vi "Process.vi"(8 "error in":errorcluster, 11 "Example Instrument":refnum<class "Instrument.FrameworkTemplate.lvclass">) -> (0 "error out":errorcluster, 3 "Example Instrument out":refnum<class "Instrument.FrameworkTemplate.lvclass">)   [LabVIEW 2019, in "Instrument.FrameworkTemplate.lvclass"]
doc: "---------------------------------------------------------------\nJKI State Machine Objects™\nhttp://jki.net/state-machine-objects/\nCopyright (C) 2005-2015, JKI <info@jki.net>\nALL RIGHTS RESERVED"
uses:
  Instrument.FrameworkTemplate.lvclass
  C:/Program Files (x86)/National Instruments/LabVIEW 2019/vi.lib/JKI/JKI SMO/SMO/SMO.lvclass
  <vilib>/JKI/JKI SMO/SMO/SMO.lvclass/SMO.ctl
  <vilib>/JKI/JKI SMO/SMO/Private/ReftoDVR--SMO.vi
  <userlib>/LevyLab/Instrument Framework/Instrument Types/VSource/Instrument.VSource.lvclass
  <vilib>/JKI/JKI SMO/SMO/SMO.lvclass
panel:
  # "Example INSTRUMENT"
  # "For instructions on how to use the JKI State Machine Objects, examples and video tutorials, visit:\nhttp://jki.net/state-machine-objects/\n\nJKI State Machine Objects™\nhttp://jki.net/state-machine-objects/\nCopyright (C) 2005-2015, JKI <info@jki.net>\nALL RIGHTS RESERVED"
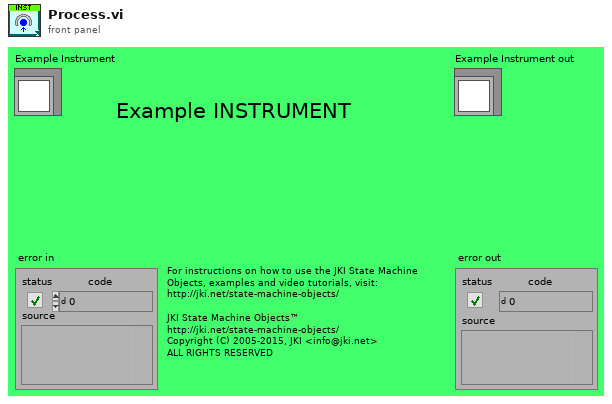
[diagram p1: front panel]
types:
  T1 = enum32{"invalid app kind", "Development System", "Run Time System", "Student Edition", "Embedded LabVIEW", "Evaluation", "Custom"}
  T2 = enum32{"Invalid", "Standard", "Closed", "Hidden", "Minimized", "Maximized"}
  T3 = enum32{"Bad", "Idle", "Run top level", "Running"}
  T4 = cluster{"Core":cluster{"Current VI Reference":refnum<vi>, "Close Panel on Exit?":bool, "error":errorcluster}, "Self Reference":refnum<class "Instrument.FrameworkTemplate.lvclass">}
  T5 = cluster{"Current VI Reference":refnum<vi>, "Close Panel on Exit?":bool, "error":errorcluster}
  T6 = typedef "SMO.lvclass/Protected Events.ctl" = cluster{"StopProcesses":refnum<user-event>, "AbortProcesses":refnum<user-event>, "Config Changed":refnum<user-event>, "Dependency":refnum<user-event>}
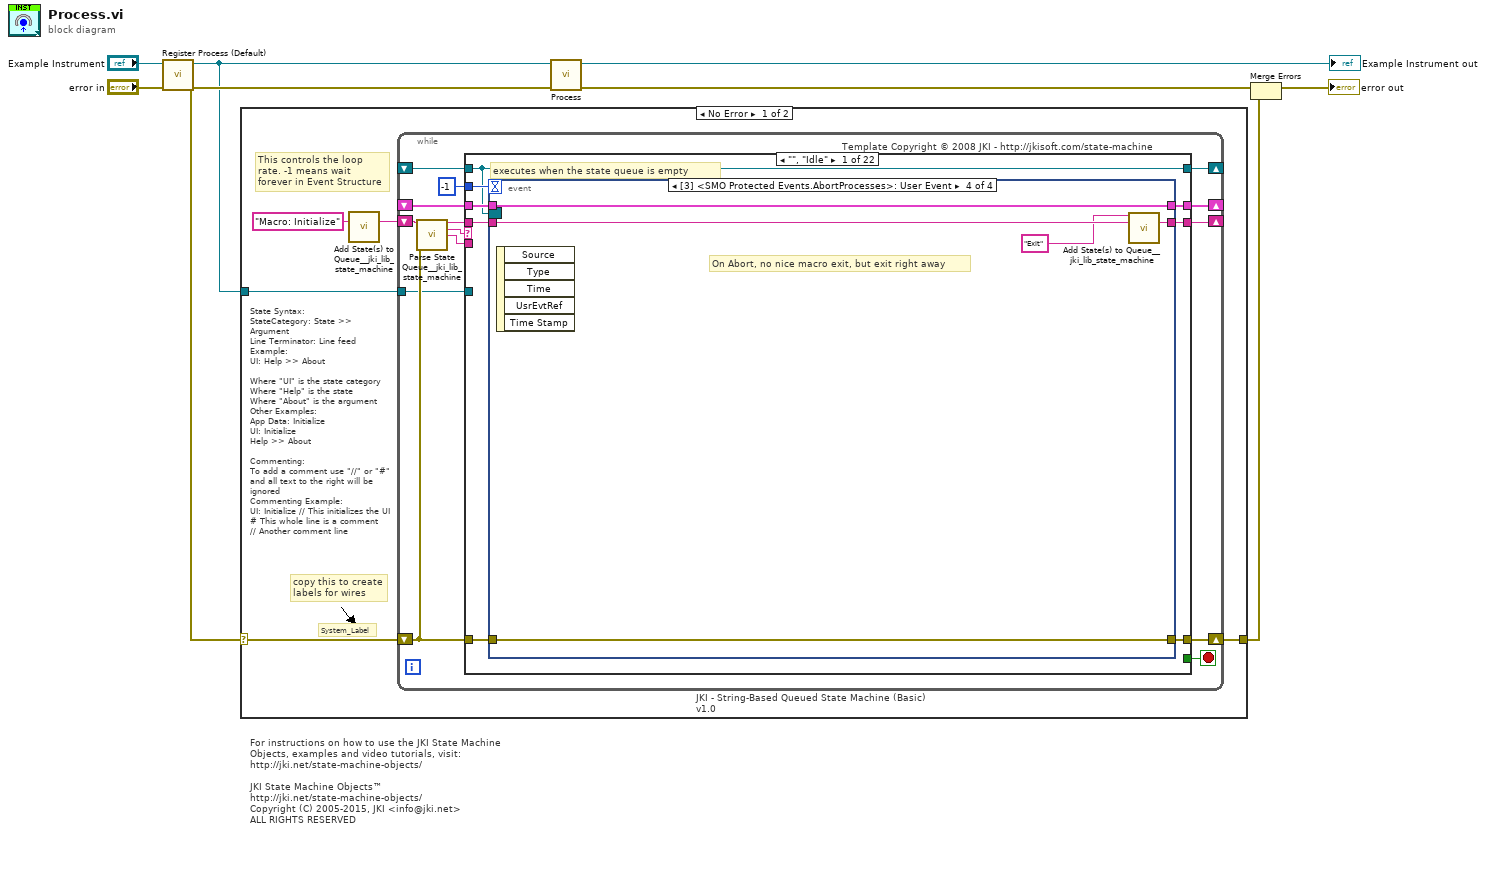
[diagram p0: block diagram]
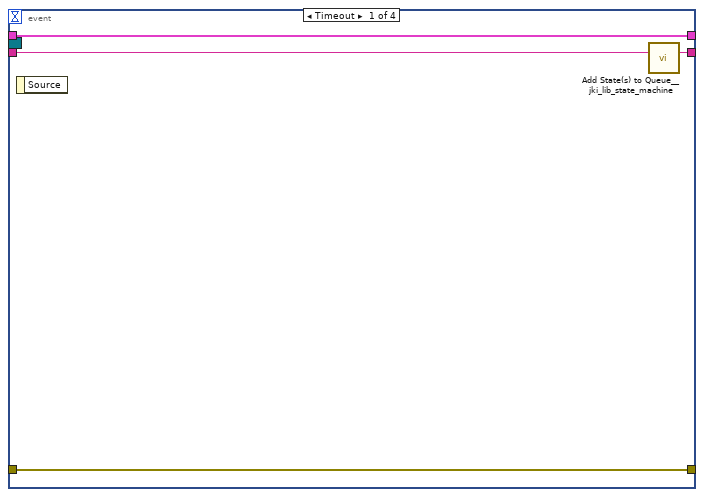
[diagram p2: hidden frame]
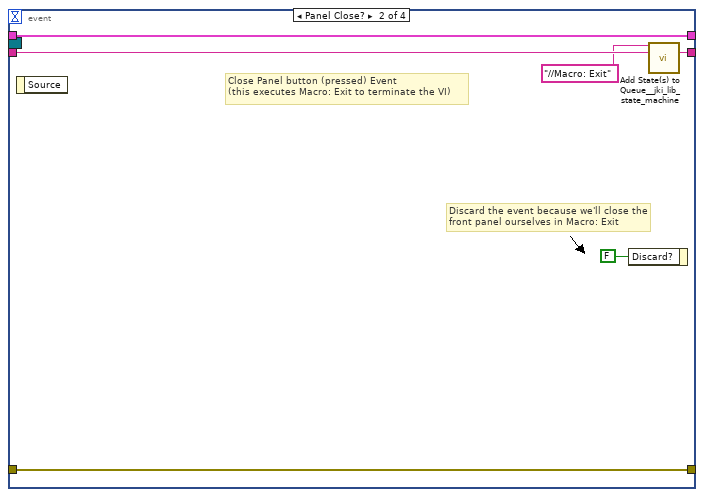
[diagram p3: hidden frame]
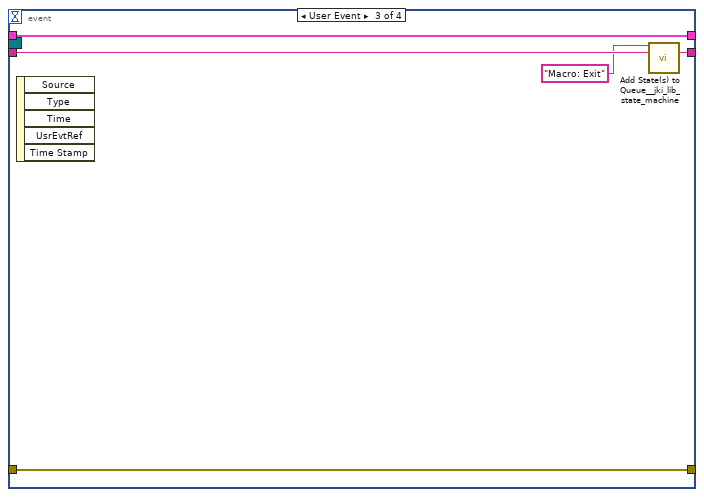
[diagram p4: hidden frame]
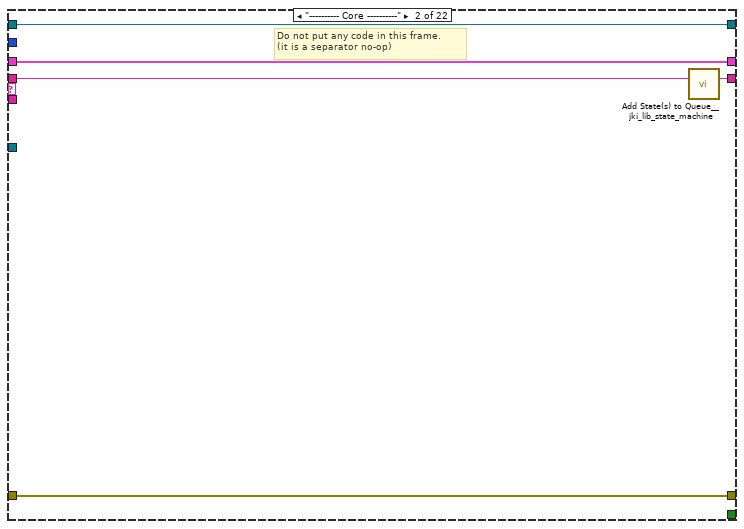
[diagram p5: hidden frame]
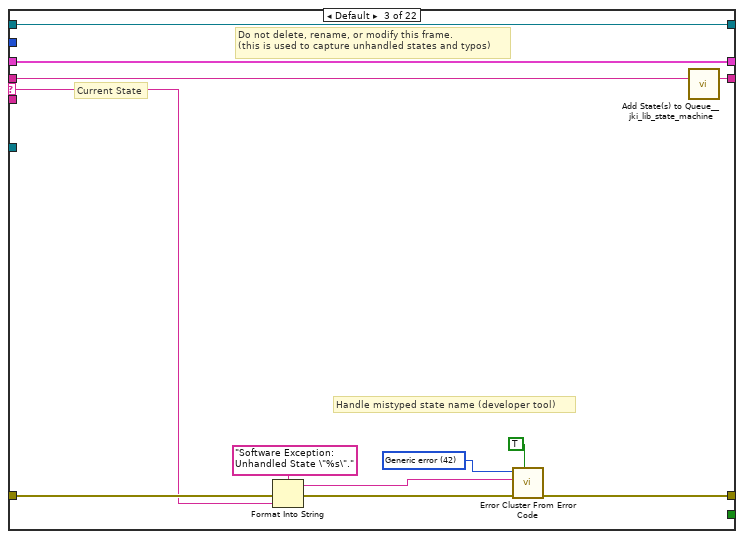
[diagram p6: hidden frame]
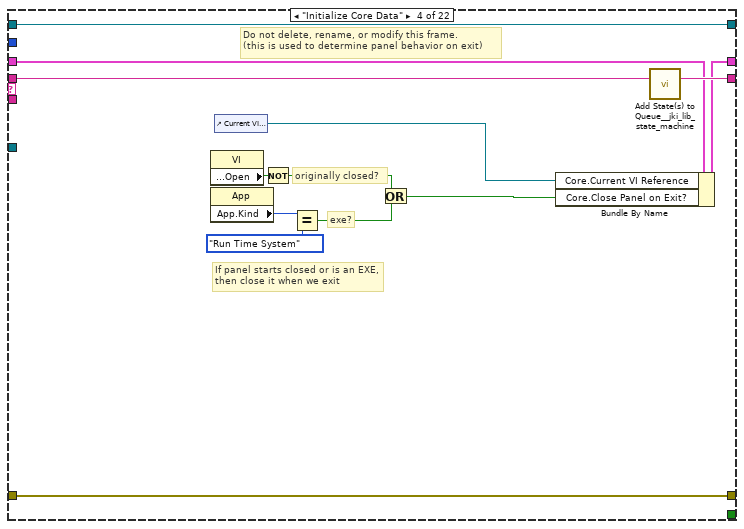
[diagram p7: hidden frame]
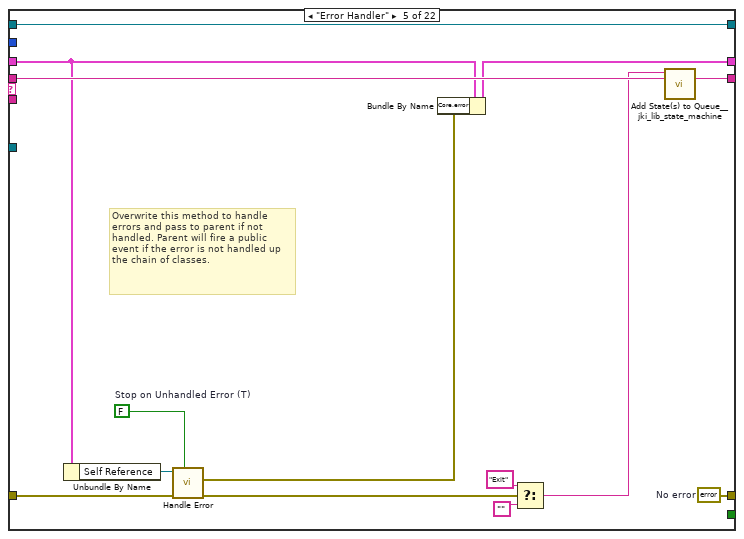
[diagram p8: hidden frame]
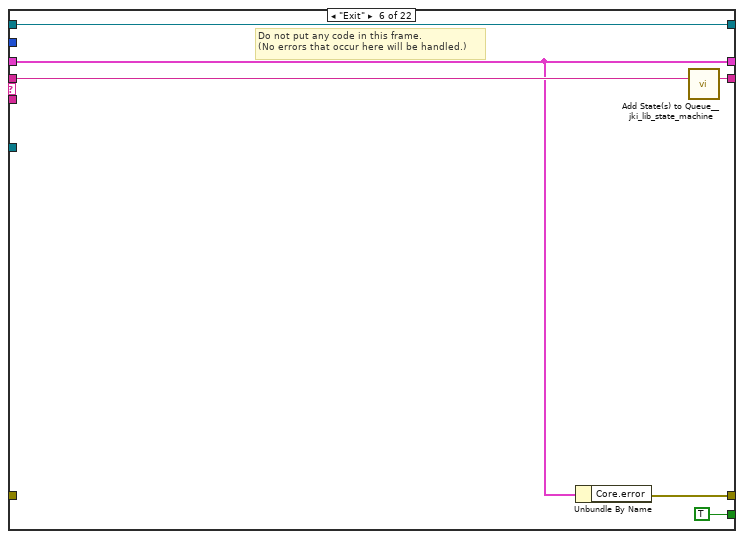
[diagram p9: hidden frame]
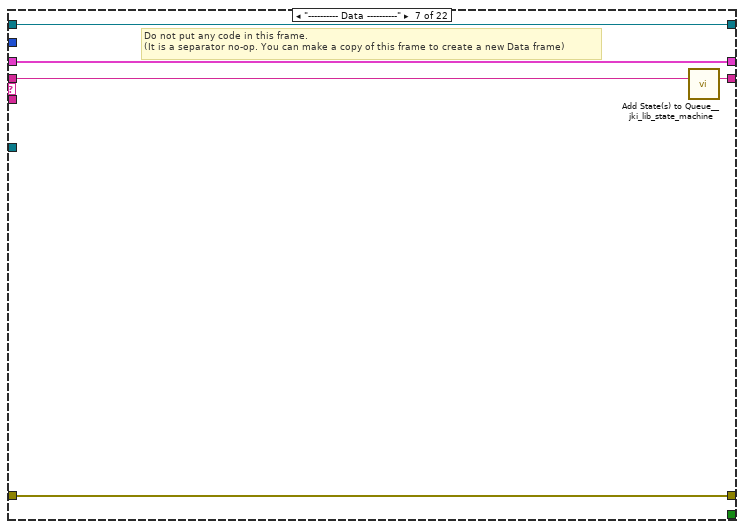
[diagram p10: hidden frame]
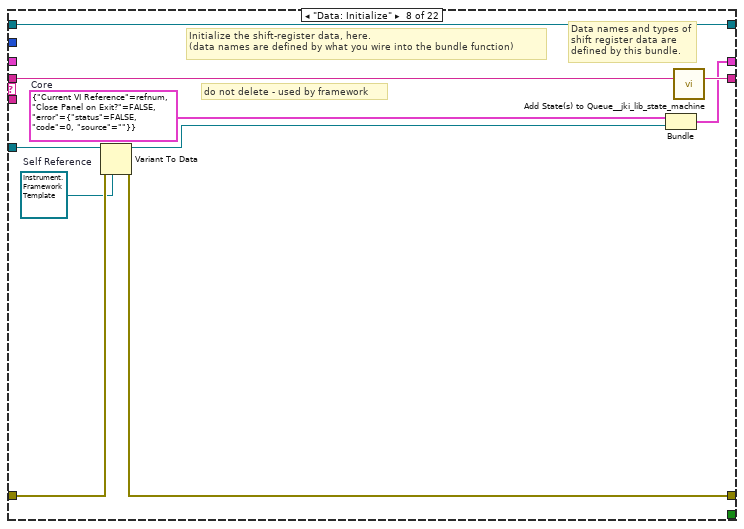
[diagram p11: hidden frame]
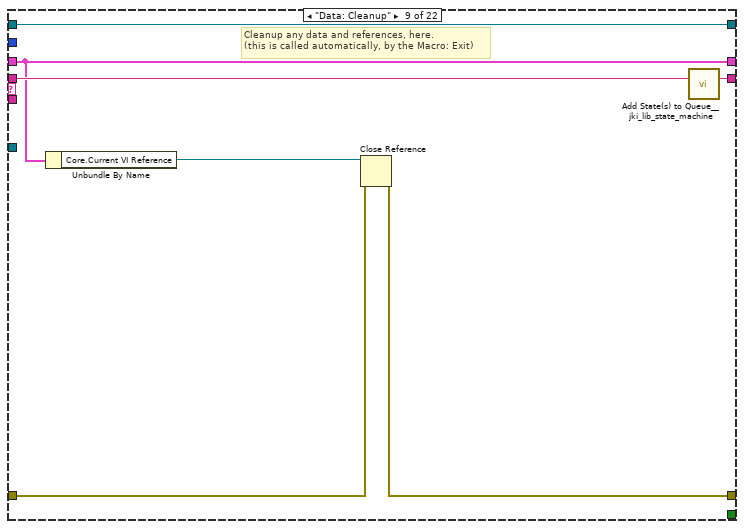
[diagram p12: hidden frame]
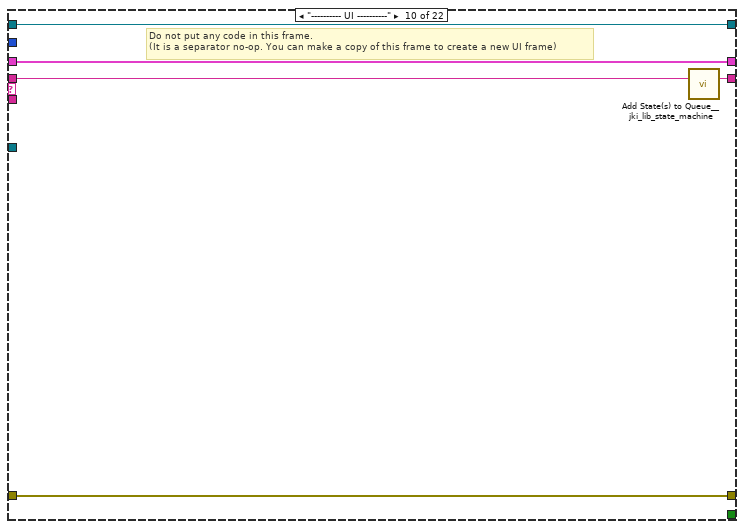
[diagram p13: hidden frame]
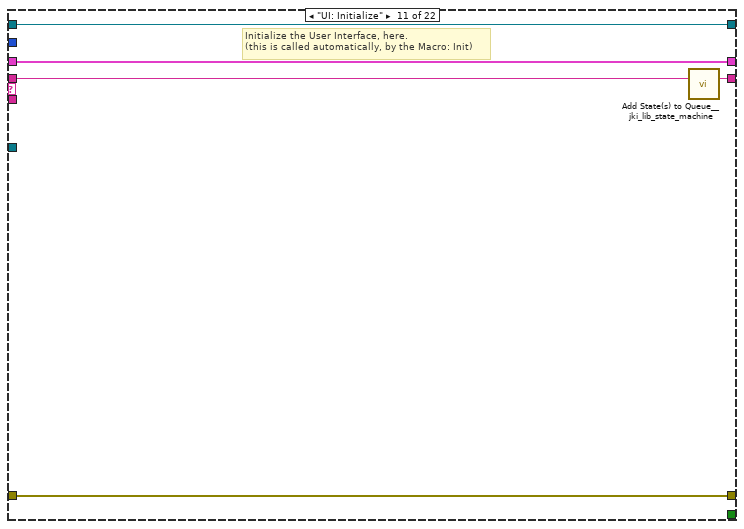
[diagram p14: hidden frame]
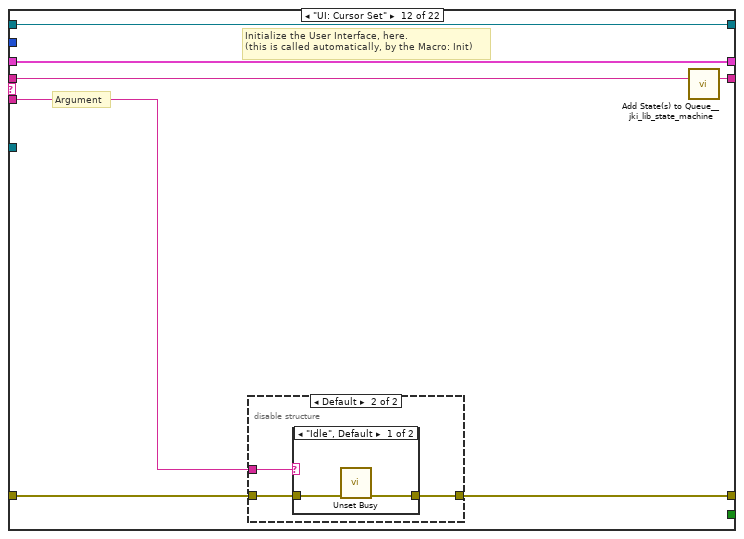
[diagram p15: hidden frame]
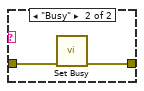
[diagram p17: hidden frame]
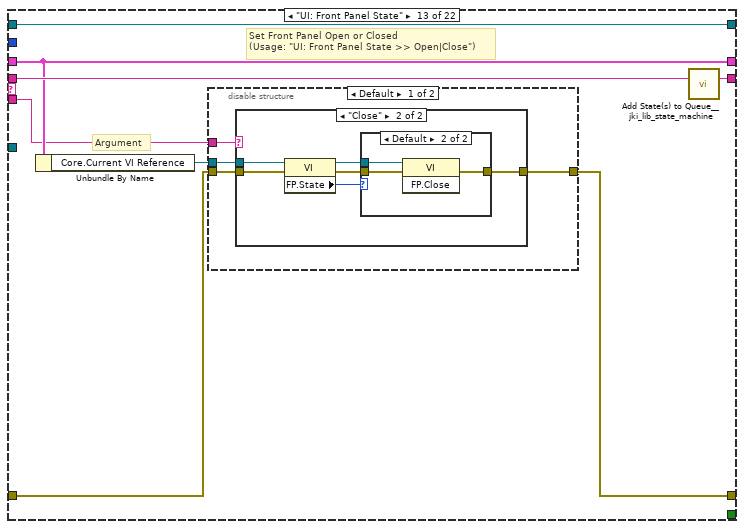
[diagram p18: hidden frame]
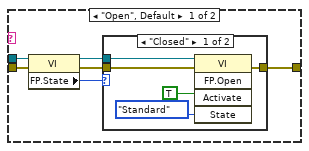
[diagram p19: hidden frame]
diagram:
  # "For instructions on how to use the JKI State Machine Objects, examples and video tutorials, visit:\nhttp://jki.net/state-machine-objects/\n\nJKI State Machine Objects™\nhttp://jki.net/state-machine-objects/\nCopyright (C) 2005-2015, JKI <info@jki.net>\nALL RIGHTS RESERVED"
  n1 = call <vilib>:"Register Process (Default).vi"("error in (no error)"="error in", "SMO"="Example Instrument") -> ("error out"=w5:errorcluster, "SelfRef"=w4:refnum<class "Instrument.FrameworkTemplate.lvclass">)  [unwired: 8 in]
  n2 = case shown="No Error" w5 {
    selector: w5 -> [w10 w279]
    tunnel: w4 -> [w11 _]
    tunnel: [w9 w279] -> w1
    frame No Error {
      # "State Syntax:\nStateCategory: State >> Argument\nLine Terminator: Line feed\nExample:\nUI: Help >> About\n\nWhere \"UI\" is the state category\nWhere \"Help\" is the state\nWhere \"About\" is the argument\nOther Examples:\nApp Data: Initialize\nUI: Initialize\nHelp >> About\n\nCommenting:\nTo add a comment use \"//\" or \"#\" and all text to the right will be ignored\nCommenting Example:\nUI: Initialize // This initializes the UI\n# This whole line is a comment\n// Another comment line"
      # "copy this to create labels for wires"
      # "This controls the loop rate. -1 means wait forever in Event Structure"
      # "System_Label"
      n3 = call <vilib>:"Add State(s) to Queue__jki_lib_state_machine.vi"("State(s) in (\"\")"="Macro: Initialize") -> ("States Out"=w13:string)  [unwired: 14 in]
      n4 = while "JKI - String-Based Queued State Machine (Basic) v1.0" {
        shift-right: [w20] -> _
        shift-left: _ -> [w19]
        shift-right: [w23] -> w9
        shift-left: w10 -> [w17]
        shift-right: [w22] -> _
        shift-left: w13 -> [w24]
        tunnel: w11 -> [w16]
        shift-right: [w15] -> _
        shift-left: _ -> [w14]
        stop <- w21 stop-if-true
        # "Template Copyright © 2008 JKI - http://jkisoft.com/state-machine"
        n5 = call <vilib>:"Parse State Queue__jki_lib_state_machine.vi"("State Queue"=w24, "Error In (no error)"=w17) -> ("Remaining States"=w26:string, "Current State"=w27:string, "Arguments"=w25:string)  [unwired: 11 in]
        n6 = case shown="\"\", \"Idle\"" w27 {
          selector: w27 -> [_ _ w62 _ _ _ _ _ _ _ _ _ _ _ _ _ _ _ _ _ _ _]
          tunnel: w26 -> [w35 w60 w66 w85 w99 w105 w110 w120 w127 w132 w137 w144 w160 w192 w215 w236 w241 w252 w257 w267 w273 w278]
          tunnel: w25 -> [_ _ _ _ _ _ _ _ _ _ _ w138 w154 _ _ _ _ _ _ _ _ _]
          tunnel: w19 -> [w33 w57 w64 w76 w93 w101 w107 _ w122 w129 w135 w142 w156 w189 w212 w217 w238 w249 w254 w258 w271 w276]
          tunnel: [w32 w58 w68 w82 w94 w100 w108 w111 w123 w130 w134 w139 w157 w190 w194 w219 w239 w243 w255 w262 w269 w274] -> w23
          tunnel: w17 -> [w31 w58 w67 w82 w95 _ w108 w117 w124 w130 w134 w140 w158 w190 w195 w220 w239 w244 w255 w263 w269 w274]
          tunnel: [w34 w59 w65 w84 w98 w104 w109 w119 w126 w131 w136 w143 w159 w191 w214 w235 w240 w251 w256 w266 w272 w277] -> w22
          tunnel: [_ _ _ _ _ TRUE _ _ _ _ _ _ _ _ _ _ _ _ _ _ _ _] -> w21
          tunnel: [w30 w57 w64 w83 w92 w101 w107 w118 w122 w129 w135 w142 w156 w189 w212 w217 w238 w249 w254 w258 w271 w276] -> w20
          tunnel: -1 ("Timeout") -> [w29 _ _ _ _ _ _ _ _ _ _ _ _ _ _ _ _ _ _ _ _ _]
          tunnel: w16 -> [_ _ _ _ _ _ _ w115 _ _ _ _ _ _ w203 w216 _ _ _ _ _ _]
          tunnel: [w28 w56 w61 w73 w97 w102 w106 w114 w121 w128 w133 w141 w153 w188 w213 w230 w237 w250 w253 w265 w270 w275] -> w15
          tunnel: w14 -> [w28 w56 w61 w73 w97 w102 w106 w114 w121 w128 w133 w141 w153 w188 w213 w230 w237 w250 w253 _ w270 w275]
          frame "", "Idle" {
            # "executes when the state queue is empty"
            n7 = event shown="[3] <SMO Protected Events.AbortProcesses>: User Event" {
              selector: w28 -> [_ _ _ _]
              dyn-events: _ -> [_ _ _ _]
              timeout: w29 -> [_ _ _ _]
              tunnel: w35 -> [w39 w45 w50 w55]
              tunnel: [w38 w44 w49 w54] -> w34
              tunnel: w33 -> [w36 w42 w47 w52]
              tunnel: [w37 w43 w48 w53] -> w32
              tunnel: w31 -> [w37 w43 w48 w53]
              tunnel: [w36 w42 w47 w52] -> w30
              event Timeout {
                n8 = event-data() -> ()  [unwired: 1 in, 1 out]
                n9 = call <vilib>:"Add State(s) to Queue__jki_lib_state_machine.vi"("State(s) in (\"\")"=w39) -> ("States Out"=w38:string)  [unwired: 14 in]
              }
              event Panel Close? {
                # "Discard the event because we'll close the front panel ourselves in Macro: Exit"
                # "Close Panel button (pressed) Event\n(this executes Macro: Exit to terminate the VI)"
                n10 = event-data() -> ()  [unwired: 1 in, 1 out]
                n11 = event-data("Discard?"=FALSE) -> ()  [unwired: 1 in, 1 out]
                n12 = call <vilib>:"Add State(s) to Queue__jki_lib_state_machine.vi"("State(s) in Front (\"\")"="//Macro: Exit", "State(s) in (\"\")"=w45) -> ("States Out"=w44:string)  [unwired: 13 in]
              }
              event User Event {
                n13 = event-data() -> ()  [unwired: 1 in, 5 out]
                n14 = call <vilib>:"Add State(s) to Queue__jki_lib_state_machine.vi"("State(s) in Front (\"\")"="Macro: Exit", "State(s) in (\"\")"=w50) -> ("States Out"=w49:string)  [unwired: 13 in]
              }
              event User Event {
                # "On Abort, no nice macro exit, but exit right away"
                n15 = event-data() -> ()  [unwired: 1 in, 5 out]
                n16 = call <vilib>:"Add State(s) to Queue__jki_lib_state_machine.vi"("State(s) in Front (\"\")"="Exit", "State(s) in (\"\")"=w55) -> ("States Out"=w54:string)  [unwired: 13 in]
              }
            }
          }
          frame "---------- Core ----------" {
            # "Do not put any code in this frame.\n(it is a separator no-op)"
            n17 = call <vilib>:"Add State(s) to Queue__jki_lib_state_machine.vi"("State(s) in (\"\")"=w60) -> ("States Out"=w59:string)  [unwired: 14 in]
          }
          frame Default {
            w71 = 42 items=["No error", "Argument error", "Memory is full", "Out of zone", "End of file", "File already open", "Generic file I/O error", "File not found", "File permission error", "Disk is full", "Duplicate path", "Too many files open", "System feature not enabled", "Resource file not found", "Cannot add resource", "Resource not found", "Image not found", "Image memory error", "Pen does not exist", "Config type invalid", "Config token not found", "Config parse error", "Config memory error", "Bad external code format", "Bad external code offset", "External code not present", "Null window", "Destroy window error", "Null menu", "Print aborted", "Bad print record", "Print driver error", "Windows error during printing", "Memory error during printing", "Print dialog error", "Generic print error", "Invalid device refnum", "Device not found", "Device parameter error", "Device unit error", "Cannot open device", "Device call aborted", "Generic error", "Cancelled by user", "Object ID too low", "Object ID too high", "Object not in heap", "Unknown heap", "Unknown object (invalid DefProc)", "Unknown object (DefProc not in table)", "Message out of range", "Invalid (null) method", "Unknown message", "Manager call not supported", "Bad address", "Network operation in progress", "Network operation timed out", "Connection is busy", "Network attribute not supported", "Network error", "Address in use", "System out of memory", "Connection aborted", "Connection refused", "Not connected", "Already connected", "Connection closed", "Initialization error (interapplication manager)", "Bad occurrence", "Wait on unbound occurrence handler", "Occurrence queue overflow", "Datalog type conflict", "Unused", "Unrecognized type (interapplication manager)", "Memory corrupt", "Failed to make temporary DLL", "Old CIN version", "Drag socket not found", "Failed to load drop-object", "Failed to register OLE object", "Failed to release OLE object", "Format specifier type mismatch", "Unknown format specifier", "Too few format specifiers", "Too many format specifiers", "Scan failed", "Newer CIN version", "Error converting to variant", "Runtime menu error", "Password tampered", "Variant attribute not found", "Incompatible variant data type", "Event data is not available", "Event Store is not present", "Occurrence is not found", "Event Queue is not created", "Event info is not available", "Refnum passed is NULL", "Error retrieving Class GUID", "Error retrieving CoClass GUID", "Error retrieving TypeLib GUID.", "Bad built application magic bytes.", "Specific driver is different from the specific driver associated with the Logical Name.", "There is no session opened to the class driver.", "Max Error", "MAX - Error with config objects", "MAX - Error loading configuration", "MAX - Group not supported"]
            # "Current State"
            # "Do not delete, rename, or modify this frame.\n(this is used to capture unhandled states and typos)"
            # "Handle mistyped state name (developer tool)"
            n18 = Format Into String(format string="Software Exception: Unhandled State \"%s\"." ("message"), error in=w67, w62) -> (resulting string=w70:string, error out=w69:errorcluster)  [unwired: 1 in]
            n19 = call <vilib>:"Error Cluster From Error Code.vi"("show call chain? (False)"=TRUE, "error in (no error)"=w69, "error message (\"\")"=w70, "error code (0)"=w71) -> ("error out"=w68:errorcluster)  [unwired: 5 in]
            n20 = call <vilib>:"Add State(s) to Queue__jki_lib_state_machine.vi"("State(s) in (\"\")"=w66) -> ("States Out"=w65:string)  [unwired: 14 in]
          }
          frame "Initialize Core Data" {
            # "Do not delete, rename, or modify this frame.\n(this is used to determine panel behavior on exit)"
            # "originally closed?"
            # "exe?"
            # "If panel starts closed or is an EXE, then close it when we exit"
            n21 = property class="VI"() -> ("Front Panel.Open"=w81:bool)  [unwired: 2 in, 2 out]
            n22 = property class="App"() -> ("App.Kind"=w80:T1)  [unwired: 2 in, 2 out]
            n23 = control-ref of="Current VI Reference"() -> (w74:refnum<vi>)
            n24 = Not(x=w81) -> (.not. x?=w78:bool)
            n25 = Equal?(x=w80, y=T1."Run Time System" ("Application:Kind")) -> (x = y?=w77:bool)
            n26 = Or(x=w78, y=w77) -> (x .or. y?=w75:bool)
            n27 = Bundle By Name(cluster=w76, "Core.Current VI Reference"=w74, "Core.Close Panel on Exit?"=w75) -> (w83:T4)
            n28 = call <vilib>:"Add State(s) to Queue__jki_lib_state_machine.vi"("State(s) in (\"\")"=w85) -> ("States Out"=w84:string)  [unwired: 14 in]
          }
          frame "Error Handler" {
            w86 = FALSE  # Stop on Unhandled Error (T)
            w94 = errorcluster {"status"=FALSE, "code"=0, "source"=""}  # No error
            # "Overwrite this method to handle errors and pass to parent if not handled. Parent will fire a public event if the error is not handled up the chain of classes."
            n29 = Unbundle By Name(w93) -> ("Self Reference"=w96:refnum<class "Instrument.FrameworkTemplate.lvclass">)
            n30 = call-dynamic "Handle Error.vi"("Stop on Unhandled Error (T)"=w86, "error in"=w95, "SMO"=w96) -> ("handling error"=w87:errorcluster, "Unhandled error"=w90:errorcluster)  [unwired: 6 in, 1 out]
            n31 = Bundle By Name(cluster=w93, "Core.error"=w90) -> (w92:T4)
            n32 = Select(t="Exit", s=w87, f="") -> (s? t:f=w91:string)
            n33 = call <vilib>:"Add State(s) to Queue__jki_lib_state_machine.vi"("State(s) in Front (\"\")"=w91, "State(s) in (\"\")"=w99) -> ("States Out"=w98:string)  [unwired: 13 in]
          }
          frame "Exit" {
            # "Do not put any code in this frame.\n(No errors that occur here will be handled.)"
            n34 = Unbundle By Name(w101) -> ("Core.error"=w100:errorcluster)
            n35 = call <vilib>:"Add State(s) to Queue__jki_lib_state_machine.vi"("State(s) in (\"\")"=w105) -> ("States Out"=w104:string)  [unwired: 14 in]
          }
          frame "---------- Data ----------" {
            # "Do not put any code in this frame.\n(It is a separator no-op. You can make a copy of this frame to create a new Data frame)"
            n36 = call <vilib>:"Add State(s) to Queue__jki_lib_state_machine.vi"("State(s) in (\"\")"=w110) -> ("States Out"=w109:string)  [unwired: 14 in]
          }
          frame "Data: Initialize" {
            w113 = T5 {"Current VI Reference"=refnum, "Close Panel on Exit?"=FALSE, "error"={"status"=FALSE, "code"=0, "source"=""}}  # Core
            w116 = refnum<class "Instrument.FrameworkTemplate.lvclass"> refnum  # Self Reference
            # "do not delete - used by framework"
            # "Data names and types of shift register data are defined by this bundle."
            # "Initialize the shift-register data, here.\n(data names are defined by what you wire into the bundle function)"
            n37 = Variant To Data(error in=w117, type=w116, Variant=w115) -> (data=w112:refnum<class "Instrument.FrameworkTemplate.lvclass">, error out=w111:errorcluster)
            n38 = Bundle("Core"=w113, "Self Reference"=w112) -> (w118:T4)  [unwired: 1 in]
            n39 = call <vilib>:"Add State(s) to Queue__jki_lib_state_machine.vi"("State(s) in (\"\")"=w120) -> ("States Out"=w119:string)  [unwired: 14 in]
          }
          frame "Data: Cleanup" {
            # "Cleanup any data and references, here.\n(this is called automatically, by the Macro: Exit)"
            n40 = Unbundle By Name(w122) -> ("Core.Current VI Reference"=w125:refnum<vi>)
            n41 = Close Reference(reference=w125, error in (no error)=w124) -> (error out=w123:errorcluster)
            n42 = call <vilib>:"Add State(s) to Queue__jki_lib_state_machine.vi"("State(s) in (\"\")"=w127) -> ("States Out"=w126:string)  [unwired: 14 in]
          }
          frame "---------- UI ----------" {
            # "Do not put any code in this frame.\n(It is a separator no-op. You can make a copy of this frame to create a new UI frame)"
            n43 = call <vilib>:"Add State(s) to Queue__jki_lib_state_machine.vi"("State(s) in (\"\")"=w132) -> ("States Out"=w131:string)  [unwired: 14 in]
          }
          frame "UI: Initialize" {
            # "Initialize the User Interface, here.\n(this is called automatically, by the Macro: Init)"
            n44 = call <vilib>:"Add State(s) to Queue__jki_lib_state_machine.vi"("State(s) in (\"\")"=w137) -> ("States Out"=w136:string)  [unwired: 14 in]
          }
          frame "UI: Cursor Set" {
            # "Argument"
            # "Initialize the User Interface, here.\n(this is called automatically, by the Macro: Init)"
            n45 = disable-structure shown="Default" {
              disable-tunnel: w140 -> [w145 w148]
              disable-tunnel: [w145 w147] -> w139
              disable-tunnel: w138 -> [_ w146]
              frame condition #0 {
              }
              frame condition #1 (active) {
                n46 = case shown="\"Idle\", Default" w146 {
                  tunnel: w148 -> [w150 w152]
                  tunnel: [w149 w151] -> w147
                  frame "Idle", Default {
                    n47 = call <vilib>:"Unset Busy.vi"("error in (no error)"=w150) -> ("error out"=w149:errorcluster)  [unwired: 10 in]
                  }
                  frame "Busy" {
                    n48 = call <vilib>:"Set Busy.vi"("error in (no error)"=w152) -> ("error out"=w151:errorcluster)  [unwired: 9 in, 1 out]
                  }
                }
              }
            }
            n49 = call <vilib>:"Add State(s) to Queue__jki_lib_state_machine.vi"("State(s) in (\"\")"=w144) -> ("States Out"=w143:string)  [unwired: 14 in]
          }
          frame "UI: Front Panel State" {
            # "Argument"
            # "Set Front Panel Open or Closed\n(Usage: \"UI: Front Panel State >> Open|Close\")"
            n50 = Unbundle By Name(w156) -> ("Core.Current VI Reference"=w155:refnum<vi>)
            n51 = disable-structure shown="Default" {
              disable-tunnel: w158 -> [w164 w187]
              disable-tunnel: [w163 w187] -> w157
              disable-tunnel: w155 -> [w162 _]
              disable-tunnel: w154 -> [w161 _]
              frame condition #0 (active) {
                n52 = case shown="\"Close\"" w161 {
                  tunnel: w164 -> [w168 w181]
                  tunnel: [w170 w182] -> w163
                  tunnel: w162 -> [w169 w179]
                  frame "Open", Default {
                    n53 = property class="VI"(reference=w169, error in=w168) -> (reference out=w166:refnum<vi>, error out=w167:errorcluster, "FP.State"=w165:T2)
                    n54 = case shown="\"Closed\"" w165 {
                      tunnel: [w173 w176] -> w170
                      tunnel: w167 -> [w172 w176]
                      tunnel: w166 -> [w171 _]
                      frame "Closed" {
                        n55 = invoke class="VI" method="FP.Open"(reference=w171, error in=w172, "Activate"=TRUE, "State"=T2."Standard") -> (error out=w173:errorcluster)  [unwired: 1 in, 4 out]
                      }
                      frame Default {
                      }
                    }
                  }
                  frame "Close" {
                    n56 = property class="VI"(reference=w179, error in=w181) -> (reference out=w178:refnum<vi>, error out=w180:errorcluster, "FP.State"=w177:T2)
                    n57 = case shown="Default" w177 {
                      tunnel: [w183 w186] -> w182
                      tunnel: w180 -> [w183 w185]
                      tunnel: w178 -> [_ w184]
                      frame "Invalid", "Closed" {
                      }
                      frame Default {
                        n58 = invoke class="VI" method="FP.Close"(reference=w184, error in=w185) -> (error out=w186:errorcluster)  [unwired: 1 in, 2 out]
                      }
                    }
                  }
                }
              }
              frame condition #1 {
              }
            }
            n59 = call <vilib>:"Add State(s) to Queue__jki_lib_state_machine.vi"("State(s) in (\"\")"=w160) -> ("States Out"=w159:string)  [unwired: 14 in]
          }
          frame "---------- Macro ----------" {
            # "Do not put any code in this frame.\n(It is a separator no-op. You can make a copy of this frame to create a new Macro frame)"
            n60 = call <vilib>:"Add State(s) to Queue__jki_lib_state_machine.vi"("State(s) in (\"\")"=w192) -> ("States Out"=w191:string)  [unwired: 14 in]
          }
          frame "Macro: Initialize" {
            w204 = "Process: Sync"
            # "Initialization Macro\n(This is called once, when the VI starts)"
            n61 = control-ref of="This VI"() -> (w206:refnum<vi>)
            n62 = property class="VI"(reference=w206) -> ("Exec.State"=w205:T3)  [unwired: 1 in, 2 out]
            n63 = call-dynamic "Read Debug Mode.vi"("error in (no error)"=w195, "Instrument in"=w203) -> ("error out"=w194:errorcluster, "Debug Mode?"=w196:bool)  [unwired: 7 in, 1 out]
            n64 = Equal?(x=w205, y=T3."Run top level") -> (x = y?=w210:bool)
            n65 = Select(t="Open", s=w196, f="Close") -> (s? t:f=w201:string)
            n66 = call <vilib>:"Build State String with Arguments__JKI_lib_State_Machine.vi"("Arguments (\"\")"=w201, "State"="UI: Front Panel State") -> ("State with Arguments"=w198:string)  [unwired: 4 in]
            n67 = Select(t=w204, s=w210, f="") -> ()  [unwired: 1 out]
            n68 = call <vilib>:"Add State(s) to Queue__jki_lib_state_machine.vi"("State(s) in Front (\"\")"="UI: Initialize", "State(s) in (\"\")"=w198) -> ("States Out"=w193:string)  [unwired: 13 in]
            n69 = call <vilib>:"Add State(s) to Queue__jki_lib_state_machine.vi"("State(s) in Front (\"\")"="Data: Initialize\nInitialize Core Data\nEvents: Register", "State(s) in (\"\")"=w204, "State(s) at Back (\"\")"=w193) -> ("States Out"=w207:string)  [unwired: 12 in]
            n70 = call <vilib>:"Add State(s) to Queue__jki_lib_state_machine.vi"("State(s) in Front (\"\")"=w207, "State(s) in (\"\")"=w215) -> ("States Out"=w214:string)  [unwired: 13 in]
          }
          frame "Macro: Exit" {
            # "Exit Macro\n(This is called once, when the VI exits)"
            n71 = Unbundle By Name(w217) -> ("Core.Close Panel on Exit?"=w234:bool)
            n72 = call-dynamic "Read Debug Mode.vi"("error in (no error)"=w220, "Instrument in"=w216) -> ("error out"=w219:errorcluster, "Debug Mode?"=w218:bool)  [unwired: 7 in, 1 out]
            n73 = Select(t="Open", s=w218, f="Close") -> (s? t:f=w224:string)
            n74 = call <vilib>:"Build State String with Arguments__JKI_lib_State_Machine.vi"("Arguments (\"\")"=w224, "State"="UI: Front Panel State") -> ("State with Arguments"=w221:string)  [unwired: 4 in]
            n75 = Select(t=w221, s=w234, f="") -> (s? t:f=w232:string)
            n76 = call <vilib>:"Add State(s) to Queue__jki_lib_state_machine.vi"("State(s) in Front (\"\")"="Data: Cleanup\nEvents: Unregister", "State(s) in (\"\")"="Process: Sync", "State(s) at Back (\"\")"="Exit") -> ("States Out"=w227:string)  [unwired: 12 in]
            n77 = call <vilib>:"Add State(s) to Queue__jki_lib_state_machine.vi"("State(s) in (\"\")"=w232, "State(s) at Back (\"\")"=w227) -> ("States Out"=w231:string)  [unwired: 13 in]
            n78 = call <vilib>:"Add State(s) to Queue__jki_lib_state_machine.vi"("State(s) in Front (\"\")"=w231, "State(s) in (\"\")"=w236) -> ("States Out"=w235:string)  [unwired: 13 in]
          }
          frame "---------- Process ----------" {
            # "Template Separator\n(You can make a copy of, or modify, this frame)"
            n79 = call <vilib>:"Add State(s) to Queue__jki_lib_state_machine.vi"("State(s) in (\"\")"=w241) -> ("States Out"=w240:string)  [unwired: 14 in]
          }
          frame "Process: Sync" {
            n80 = Unbundle By Name(w249) -> ("Self Reference"=w245:refnum<class "Instrument.FrameworkTemplate.lvclass">)
            n81 = call <vilib>:"WaitOnProcessSync.vi"("error in (no error)"=w244, "SMO"=w245) -> ("error out"=w243:errorcluster, "Don't run?"=w248:bool)  [unwired: 7 in, 1 out]
            n82 = Select(t="Data: Cleanup\nEvents: Unregister\nExit", s=w248, f="") -> (s? t:f=w242:string)
            n83 = call <vilib>:"Add State(s) to Queue__jki_lib_state_machine.vi"("State(s) in Front (\"\")"=w242, "State(s) in (\"\")"=w252) -> ("States Out"=w251:string)  [unwired: 13 in]
          }
          frame "---------- Events ----------" {
            # "Template Separator\n(You can make a copy of, or modify, this frame)"
            n84 = call <vilib>:"Add State(s) to Queue__jki_lib_state_machine.vi"("State(s) in (\"\")"=w257) -> ("States Out"=w256:string)  [unwired: 14 in]
          }
          frame "Events: Register" {
            # "Expand to add\nmore events"
            n85 = Unbundle By Name(w258) -> ("Self Reference"=w259:refnum<class "Instrument.FrameworkTemplate.lvclass">)
            n86 = call <vilib>:"GetProtectedEvents.vi"("SMO"=w259) -> ("error out"=w260:errorcluster, "SMO Protected Events"=w264:T6)  [unwired: 8 in, 1 out]
            n87 = register-events(w264) -> (reference out=w265:refnum<event-registration>, error out=w261:errorcluster)  [unwired: 2 in]
            n88 = Merge Errors(w263, w261, w260) -> (w262:errorcluster)
            n89 = call <vilib>:"Add State(s) to Queue__jki_lib_state_machine.vi"("State(s) in (\"\")"=w267) -> ("States Out"=w266:string)  [unwired: 14 in]
          }
          frame "Events: Unregister" {
            n90 = Unregister For Events(event registration refnum=w270, error in=w269) -> (error out=w268:errorcluster)
            n91 = call <vilib>:"Clear Errors.vi"("error in (no error)"=w268) -> ()  [unwired: 5 in, 2 out]
            n92 = call <vilib>:"Add State(s) to Queue__jki_lib_state_machine.vi"("State(s) in (\"\")"=w273) -> ("States Out"=w272:string)  [unwired: 14 in]
          }
          frame "---------- Action ----------" {
            n93 = call <vilib>:"Add State(s) to Queue__jki_lib_state_machine.vi"("State(s) in (\"\")"=w278) -> ("States Out"=w277:string)  [unwired: 14 in]
          }
        }
      }
    }
    frame Error {
    }
  }
  n94 = call-parent "Process.vi"("error in"=w5, "Instrument"=w4) -> ("error out"=w2:errorcluster, "Instrument out"=→"Example Instrument out":refnum<class "Instrument.FrameworkTemplate.lvclass">)  [unwired: 8 in]
  n95 = Merge Errors(w2, w1) -> (→"error out":errorcluster)
